vi "Update CVT.vi"(8 "error in (no error)":errorcluster, 11 "Measurement in":refnum<class "Measurement.lvclass">) -> (0 "error out":errorcluster, 3 "Measurement out":refnum<class "Measurement.lvclass">)   [LabVIEW 2017, in "Measurement Actor.lvlib" / "Measurement.lvclass"]
uses:
  Measurement.lvclass
  Hardware/Hardware.lvclass
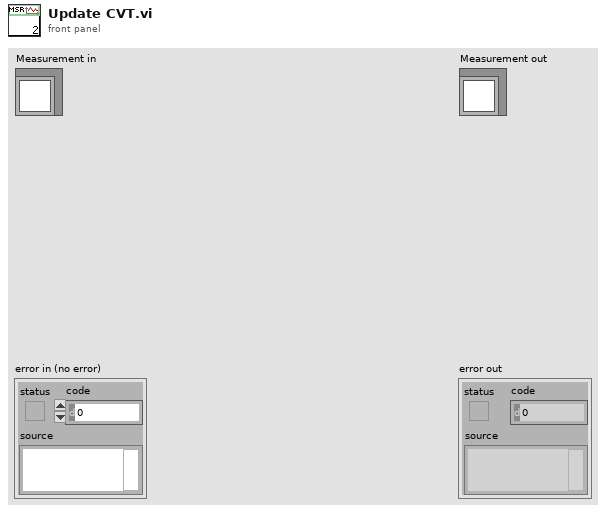
[diagram p1: front panel]
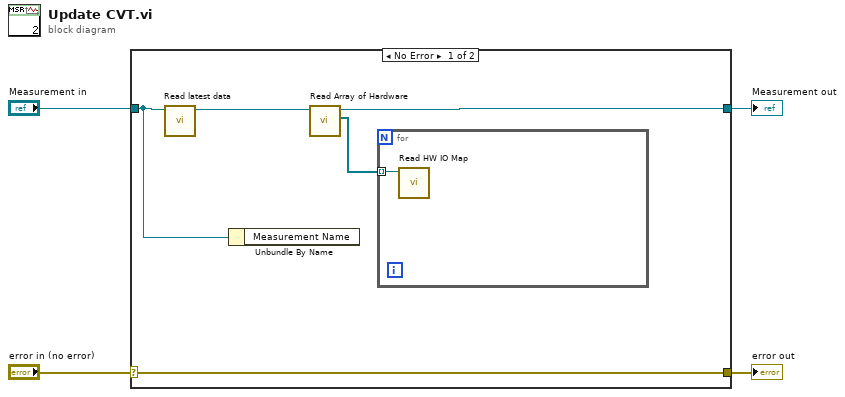
[diagram p0: block diagram]
diagram:
  n1 = case shown="No Error" "error in (no error)" {
    selector: "error in (no error)" -> [w9 w12]
    tunnel: [w9 w12] -> w3
    tunnel: [w7 w11] -> w1
    tunnel: "Measurement in" -> [w5 w11]
    frame No Error {
      n2 = call "Read latest data.vi"("Measurement in"=w5) -> ("Measurement out"=w8:refnum<class "Measurement.lvclass">)  [unwired: 8 in, 2 out]
      n3 = Unbundle By Name(w5) -> ()  [unwired: 1 out]
      n4 = call "Read Array of Hardware.vi"("Measurement in"=w8) -> ("Array of Hardware"=w6:refnum<class "Hardware.lvclass">[], "Measurement out"=w7:refnum<class "Measurement.lvclass">)  [unwired: 8 in, 1 out]
      n5 = for {
        tunnel: w6 -> [w10] mode=indexing
        n6 = call "Read HW IO Map.vi"("Hardware in"=w10) -> ()  [unwired: 8 in, 3 out]
      }
    }
    frame Error {
    }
  }
  "error out" <- w3
  "Measurement out" <- w1
